vi "rename channel.vi"(8 "error in":errorcluster, 9 "new name":string, 10 "old name":string, 11 "Scaling configuration in":refnum<class "Scaling configuration.lvclass">) -> (0 "error out":errorcluster, 3 "Scaling configuration out":refnum<class "Scaling configuration.lvclass">)   [LabVIEW 2013, in "Scaling configuration.lvclass"]
uses:
  Scaling configuration.lvclass
  <vilib>/NI/Tag Bus/tag/tag descriptor.lvclass/tag descriptor.ctl
  Scaling configuration.lvclass/Scaling configuration.ctl
  <vilib>/NI/Tag Bus Module Framework/channel/TBM channel.lvclass
  <vilib>/NI/Tag Bus/tag/tag descriptor.lvclass
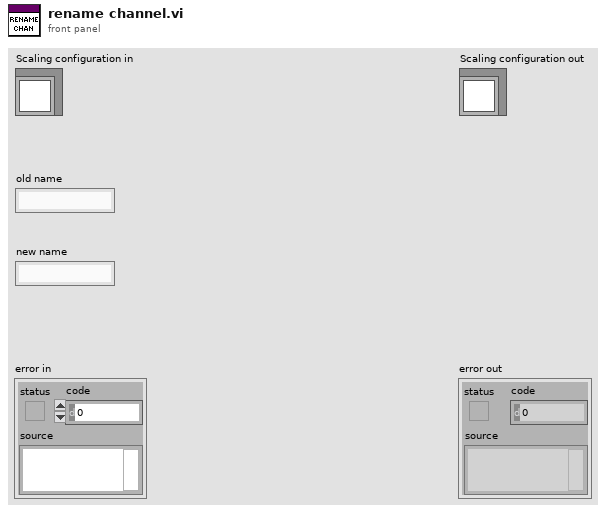
[diagram p1: front panel]
types:
  T1 = typedef "Scaling configuration.lvclass/scale data types.ctl" = enum16{"Double", "Single", "I64", "I32", "I16", "I8", "U64", "U32", "U16", "U8"}
  T2 = cluster{"mappings":cluster{"input channel":refnum<class "TBM channel.lvclass">, "output channel":refnum<class "TBM channel.lvclass">, "input data type":T1, "output data type":T1}[], "name":string}[]
  T3 = cluster{"input channel":refnum<class "TBM channel.lvclass">, "output channel":refnum<class "TBM channel.lvclass">, "input data type":T1, "output data type":T1}[]
  T4 = cluster{"input channel":refnum<class "TBM channel.lvclass">, "output channel":refnum<class "TBM channel.lvclass">, "input data type":T1, "output data type":T1}
  T5 = cluster{"mappings":cluster{"input channel":refnum<class "TBM channel.lvclass">, "output channel":refnum<class "TBM channel.lvclass">, "input data type":T1, "output data type":T1}[], "name":string}
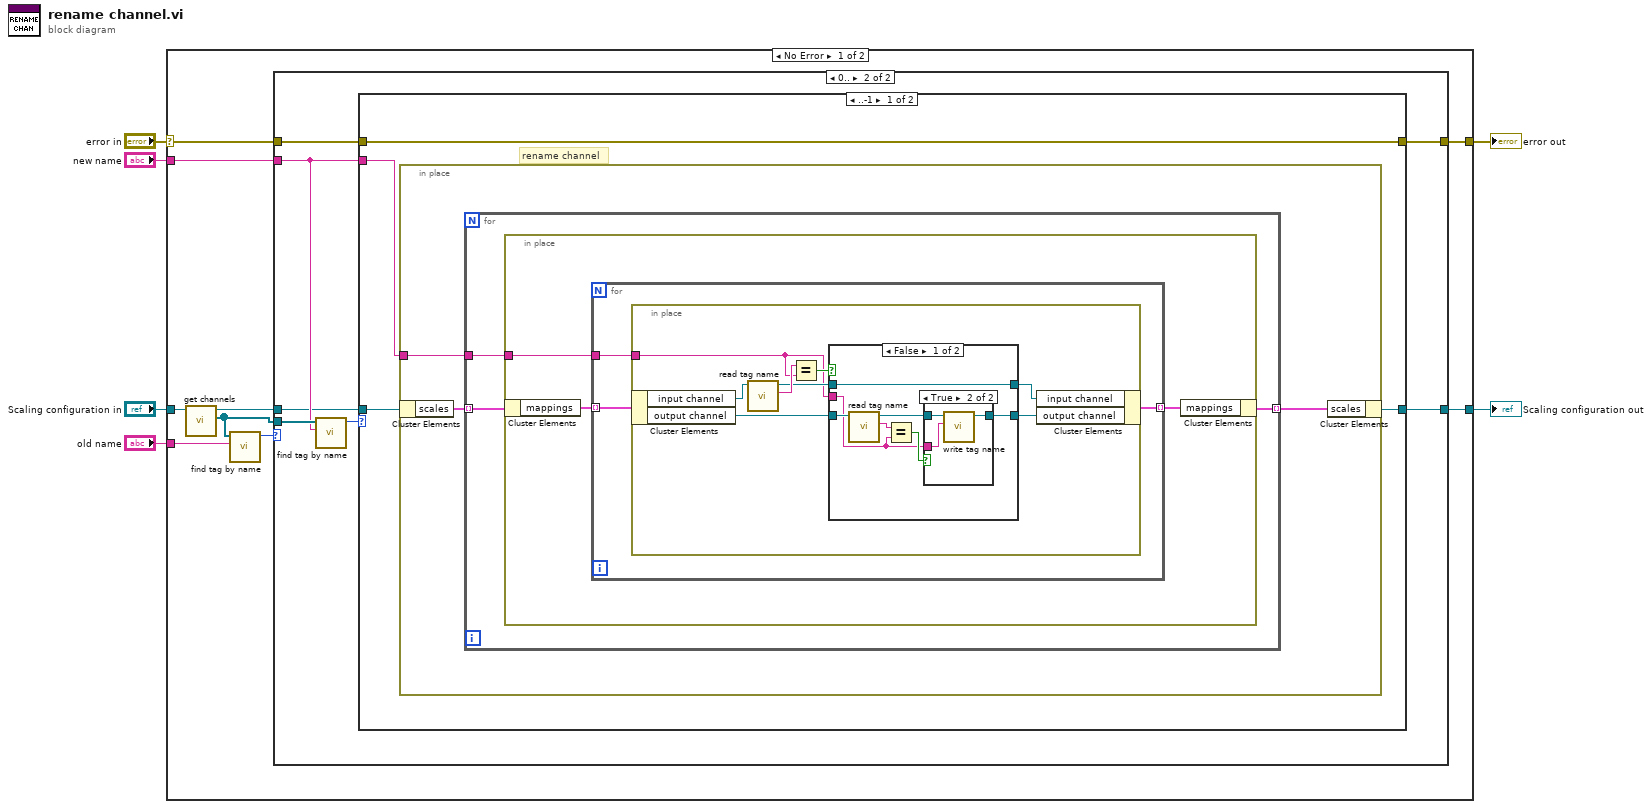
[diagram p0: block diagram]
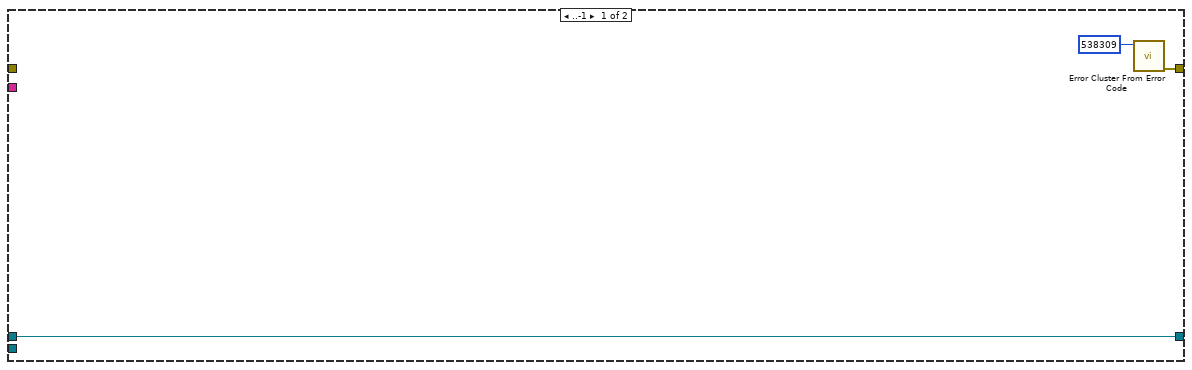
[diagram p2: hidden frame]
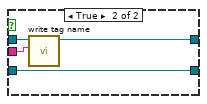
[diagram p4: hidden frame]
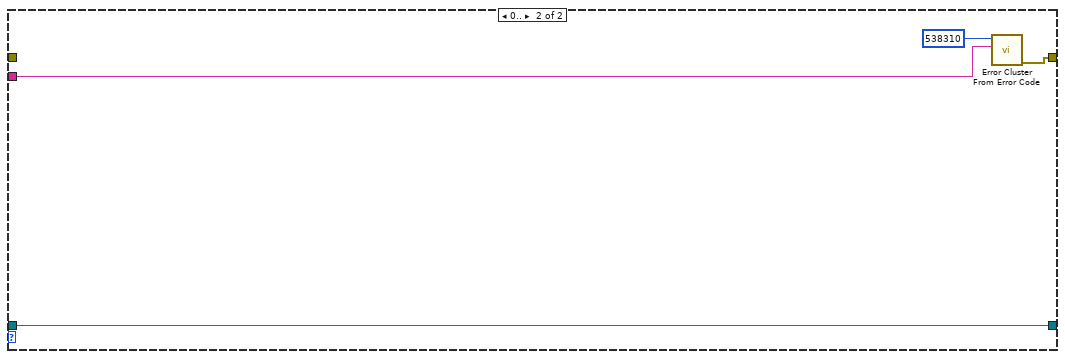
[diagram p5: hidden frame]
diagram:
  n1 = case shown="No Error" "error in" {
    selector: "error in" -> [w10 w70]
    tunnel: "new name" -> [w11 _]
    tunnel: "Scaling configuration in" -> [w15 w69]
    tunnel: [w7 w69] -> w4
    tunnel: [w9 w70] -> w3
    tunnel: "old name" -> [w14 _]
    frame No Error {
      n2 = call-dynamic "get channels.vi"("Scaling configuration in"=w15) -> ("channels"=w12:refnum<class "TBM channel.lvclass">[], "Scaling configuration out"=w8:refnum<class "Scaling configuration.lvclass">)  [unwired: 9 in]
      n3 = call <vilib>:"find tag by name.vi"("name"=w14, "tags in"=w12) -> ("index"=w13:i32)  [unwired: 9 in]
      n4 = case shown="0.." w13 {
        tunnel: w12 -> [_ w25]
        tunnel: [w17 w22] -> w9
        tunnel: w11 -> [_ w24]
        tunnel: w10 -> [_ w21]
        tunnel: w8 -> [w16 w20]
        tunnel: [w16 w19] -> w7
        frame ..-1 {
          n5 = call <vilib>:"Error Cluster From Error Code.vi"("error code (0)"=538309) -> ("error out"=w17:errorcluster)  [unwired: 8 in]
        }
        frame 0.. {
          n6 = call <vilib>:"find tag by name.vi"("name"=w24, "tags in"=w25) -> ("index"=w23:i32)  [unwired: 9 in]
          n7 = case shown="..-1" w23 {
            tunnel: w24 -> [w26 w66]
            tunnel: [w29 w68] -> w22
            tunnel: w21 -> [w29 _]
            tunnel: w20 -> [w28 w65]
            tunnel: [w27 w65] -> w19
            frame ..-1 {
              # "rename channel"
              n8 = in-place {
                in-place-border: w26 -> [w31]
                n9 = in-place-cluster #1(w28) -> ("scales"=w32:T2)
                n10 = for {
                  tunnel: w32 -> [w35] mode=indexing
                  tunnel: w31 -> [w34]
                  tunnel: [w33] -> w30 mode=indexing
                  n11 = in-place {
                    in-place-border: w34 -> [w36]
                    n12 = in-place-cluster #2(w35) -> ("mappings"=w38:T3)
                    n13 = for {
                      tunnel: w38 -> [w41] mode=indexing
                      tunnel: [w40] -> w37 mode=indexing
                      tunnel: w36 -> [w39]
                      n14 = in-place {
                        in-place-border: w39 -> [w45]
                        n15 = in-place-cluster #3(w41) -> ("input channel"=w49:refnum<class "TBM channel.lvclass">, "output channel"=w43:refnum<class "TBM channel.lvclass">)
                        n16 = call <vilib>:"read tag name.vi"("system tag in"=w49) -> ("name"=w48:string, "system tag out"=w46:refnum<class "TBM channel.lvclass">)  [unwired: 8 in, 1 out]
                        n17 = Equal?(x=w48, y=w45) -> (x = y?=w47:bool)
                        n18 = case shown="False" w47 {
                          tunnel: w46 -> [w56 w64]
                          tunnel: w45 -> [w51 w63]
                          tunnel: [w56 w62] -> w44
                          tunnel: w43 -> [w55 w61]
                          tunnel: [w50 w61] -> w42
                          frame False {
                            n19 = call <vilib>:"read tag name.vi"("system tag in"=w55) -> ("name"=w54:string, "system tag out"=w52:refnum<class "TBM channel.lvclass">)  [unwired: 8 in, 1 out]
                            n20 = Equal?(x=w54, y=w51) -> (x = y?=w53:bool)
                            n21 = case shown="True" w53 {
                              tunnel: w52 -> [w57 w60]
                              tunnel: w51 -> [_ w59]
                              tunnel: [w57 w58] -> w50
                              frame False {
                              }
                              frame True {
                                n22 = call <vilib>:"write tag name.vi"("name"=w59, "system tag in"=w60) -> ("system tag out"=w58:refnum<class "TBM channel.lvclass">)  [unwired: 8 in, 1 out]
                              }
                            }
                          }
                          frame True {
                            n23 = call <vilib>:"write tag name.vi"("name"=w63, "system tag in"=w64) -> ("system tag out"=w62:refnum<class "TBM channel.lvclass">)  [unwired: 8 in, 1 out]
                          }
                        }
                        n24 = in-place-cluster #3("input channel"=w44, "output channel"=w42) -> (w40:T4)
                      }
                    }
                    n25 = in-place-cluster #2("mappings"=w37) -> (w33:T5)
                  }
                }
                n26 = in-place-cluster #1("scales"=w30) -> (w27:refnum<class "Scaling configuration.lvclass">)
              }
            }
            frame 0.. {
              n27 = call <vilib>:"Error Cluster From Error Code.vi"("error message (\"\")"=w66, "error code (0)"=538310) -> ("error out"=w68:errorcluster)  [unwired: 7 in]
            }
          }
        }
      }
    }
    frame Error {
    }
  }
  "error out" <- w3
  "Scaling configuration out" <- w4
